vi "con_sub_tec_data_v2.vi"(3 "file path":path=path "C:/luminartech/ManufacturingTools/TS_Automation/Programs/Labview/bring_up/con_sub_tec/con_sub_tec_resp.txt") -> (1 "data array":dbl[](array[numeric]))   [LabVIEW 2018]
panel:
  out "size(s)":i32
  out "data table":dbl[][](array[numeric])
  out "line":string
  out "text 2":string[](array[string])
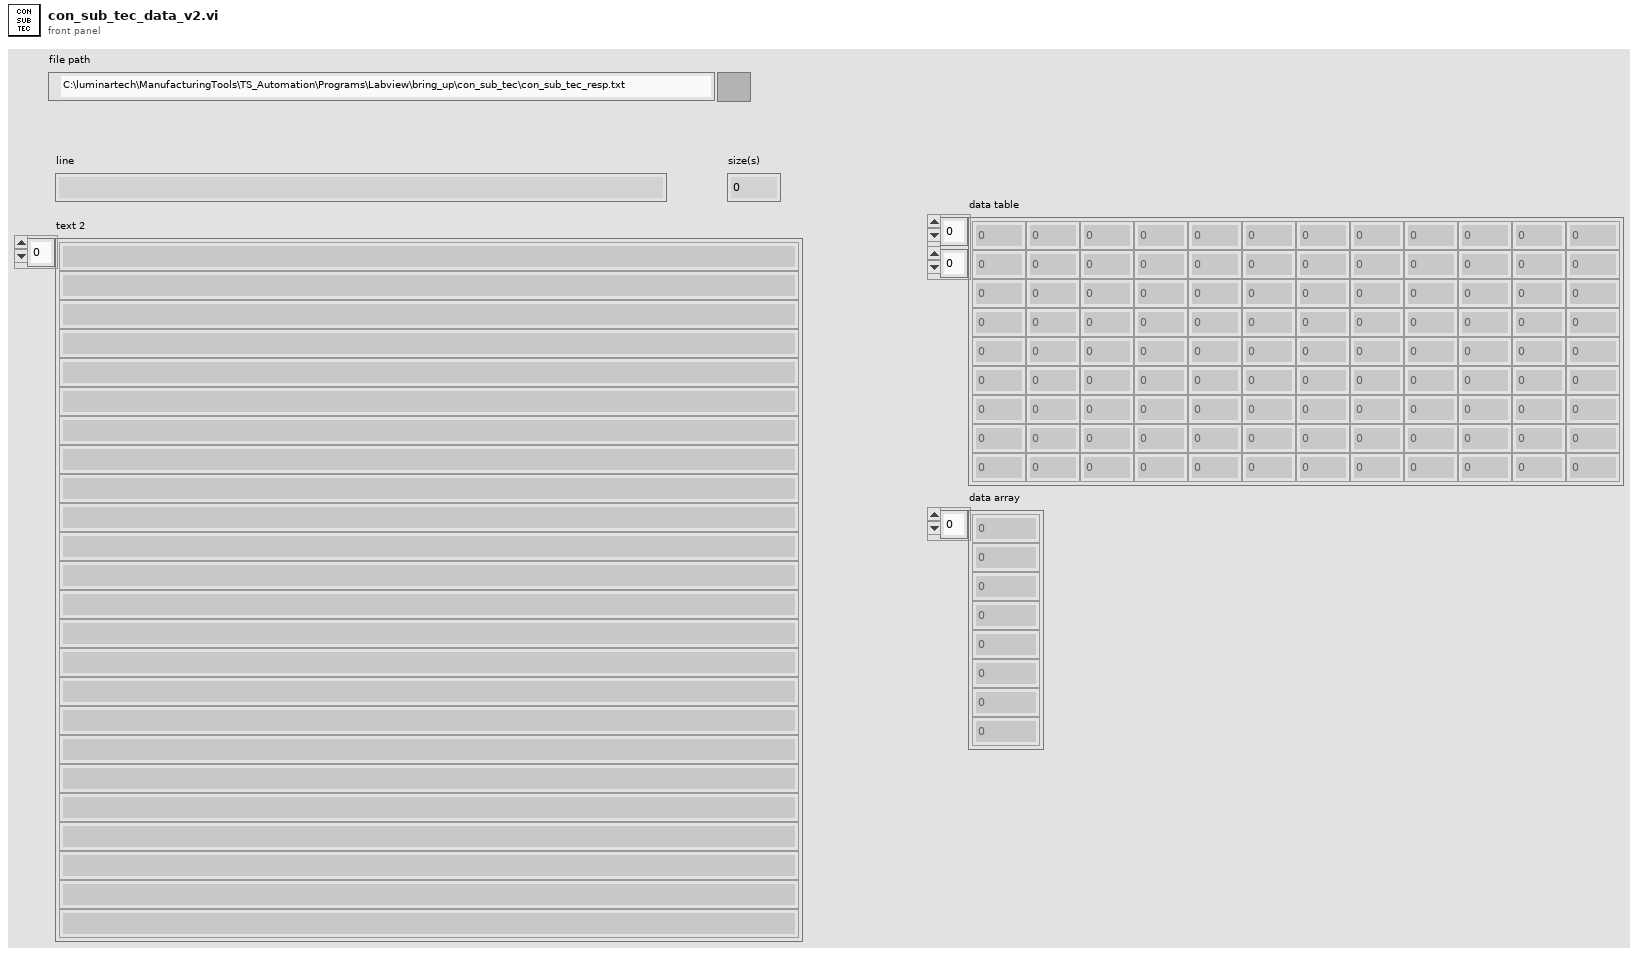
[diagram p1: front panel]
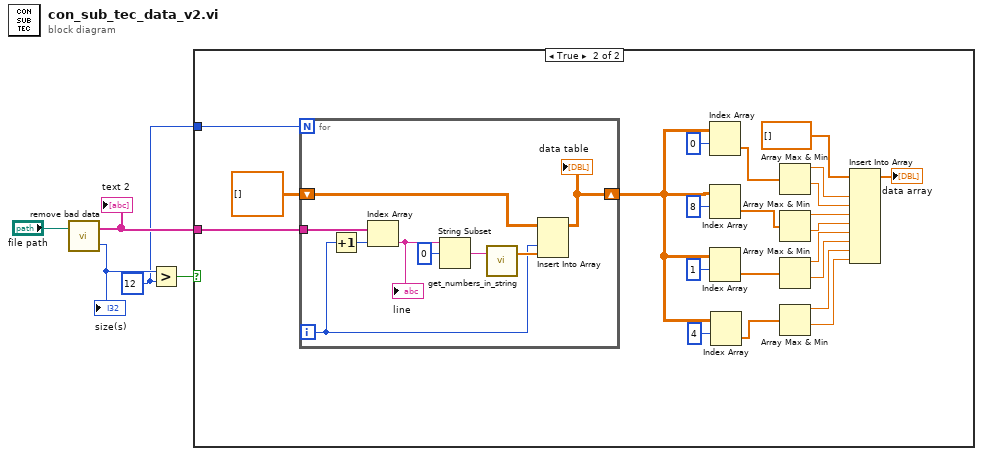
[diagram p0: block diagram]
diagram:
  w1 = 12 ("y")
  n1 = call "remove bad data.vi"("file path"="file path") -> ("size(s)"=w2:i32, "text 2"=w3:string[])  [unwired: 1 in]
  "text 2" <- w3
  "size(s)" <- w2
  n2 = Greater?(x=w2, y=w1) -> (0:w4:bool)
  n3 = case shown="True" w4 {
    tunnel: w3 -> [_ w7]
    tunnel: w1 -> [_ w6]
    frame False {
    }
    frame True {
      n4 = for {
        N: w6 -> [_]
        shift-right: [w32] -> w8
        shift-left: dbl[][] [] -> [w33]
        tunnel: w7 -> [w29]
        i -> [w30]
        n5 = Increment(x=w30) -> (x+1=w36:i32)
        n6 = Index Array(array=w29, index=w36) -> (element=w35:string)
        "line" <- w35
        n7 = String Subset(string=w35, offset (0)=0) -> (substring=w34:string)  [unwired: 1 in]
        n8 = call "get_numbers_in_string.vi"("String"=w34) -> ("Extracted Numbers"=w31:dbl[])  [unwired: 1 in, 1 out]
        n9 = Insert Into Array(array=w33, index (col)=w30, new element=w31) -> (w32:dbl[][])  [unwired: 1 in]
        "data table" <- w32
      }
      n10 = Index Array(array=w8, index (row)=0) -> (element=w26:dbl[])  [unwired: 1 in]
      n11 = Index Array(array=w8, index (row)=8) -> (element=w24:dbl[])  [unwired: 1 in]
      n12 = Index Array(array=w8, index (row)=1) -> (element=w22:dbl[])  [unwired: 1 in]
      n13 = Index Array(array=w8, index (row)=4) -> (element=w20:dbl[])  [unwired: 1 in]
      n14 = Array Max & Min(array=w26) -> (max value=w18:dbl, min value=w17:dbl)  [unwired: 2 out]
      n15 = Array Max & Min(array=w24) -> (max value=w16:dbl, min value=w15:dbl)  [unwired: 2 out]
      n16 = Array Max & Min(array=w22) -> (max value=w14:dbl, min value=w11:dbl)  [unwired: 2 out]
      n17 = Array Max & Min(array=w20) -> (max value=w10:dbl, min value=w9:dbl)  [unwired: 2 out]
      n18 = Insert Into Array(array=dbl[] [], new element #1=w18, new element #2=w17, new element #3=w16, new element #4=w15, new element #5=w14, new element #6=w11, new element #7=w10, new element #8=w9) -> (→"data array":dbl[])  [unwired: 1 in]
    }
  }
